vi "get_type.vi"(0 "MoAgSy_Message.lvclass in":refnum<class "MoAgSy_Message.lvclass">, 5 "error in (no error)":errorcluster) -> (14 "MoAgSy_Message.lvclass out":refnum<class "MoAgSy_Message.lvclass">, 16 "type":enum16{"mobile Agent", "Visitor", "Message"}(ring), 19 "error out":errorcluster)   [LabVIEW 2009, in "MoAgSy.lvlib" / "MoAgSy_Message.lvclass"]
uses:
  MoAgSy_Message.lvclass
  MoAgSy_Message.lvclass/MoAgSy_Message.ctl
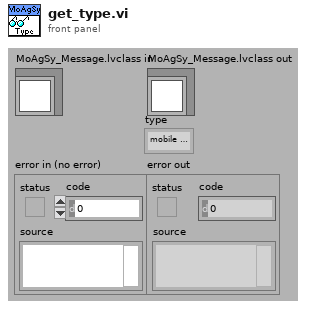
[diagram p1: front panel]
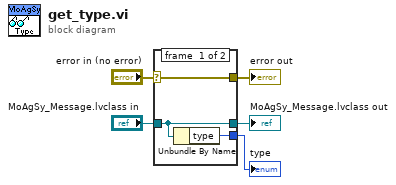
[diagram p0: block diagram]
diagram:
  n1 = case shown="No Error" "error in (no error)" {
    selector: "error in (no error)" -> [w8 w9]
    tunnel: [w8 w9] -> w4
    tunnel: [w7 w10] -> w2
    tunnel: "MoAgSy_Message.lvclass in" -> [w7 w10]
    tunnel: [w6 _] -> w1
    frame #0 {
      n2 = Unbundle By Name(w7) -> ("type"=w6:enum16{"mobile Agent", "Visitor", "Message"})
    }
    frame #1 {
    }
  }
  "error out" <- w4
  "MoAgSy_Message.lvclass out" <- w2
  "type" <- w1
